vi "UT_011_Comments.vi"() -> ()   [LabVIEW 2017]
uses:
  88135e47-21b0-4fd1-85e0-e7ee9c587d2f.vi
  lib/TOML to LabVIEW.vi
  <vilib>/addons/_JKI Toolkits/Caraya/classes/Assert/Assert True.vi
  <vilib>/addons/_JKI Toolkits/Caraya/classes/Test/Test.lvclass
  <vilib>/addons/_JKI Toolkits/Caraya/classes/Assert/Assert.lvclass
  lib/TOML.lvlib
panel:
  out "error out":errorcluster
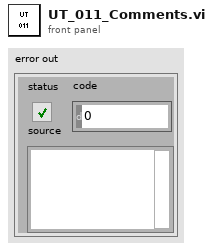
[diagram p1: front panel]
types:
  T1 = typedef "TOML.lvlib/TOML Value.ctl" = cluster{"type":enum16{"Table", "Array", "String", "Integer", "Float", "Boolean", "Offset Date-Time", "Local Date-Time", "Local Date", "Local Time", "Path"}, "value":variant}
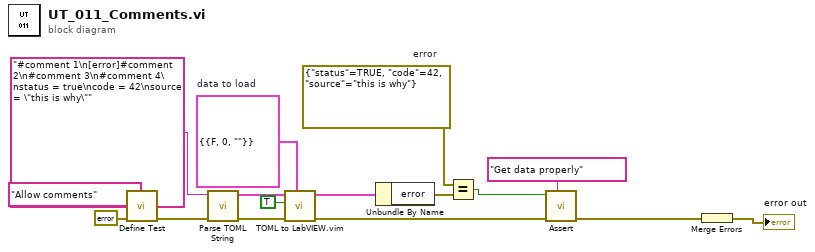
[diagram p0: block diagram]
diagram:
  w7 = cluster{"error":errorcluster} {"error"={"status"=FALSE, "code"=0, "source"=""}}  # data to load
  w9 = errorcluster {"status"=TRUE, "code"=42, "source"="this is why"}  # error
  n1 = call <vilib>:"Define Test.vi"("error in (no error)"=errorcluster {"status"=FALSE, "code"=0, "source"=""}, "Label (VI Title)"="Allow comments") -> ("error out"=w8:errorcluster)  [unwired: 9 in]
  n2 = call "Parse TOML String.vi"("error in (no error)"=w8, "String"="#comment 1\n[error]#comment 2\n#comment 3\n#comment 4\nstatus = true\ncode = 42\nsource = \"this is why\"") -> ("error out"=w2:errorcluster, "Value"=w3:T1)  [unwired: 8 in]
  n3 = call "TOML to LabVIEW.vim"("datatype"=w7, "error in (no error)"=w2, "Error if missing element"=TRUE, "Value"=w3) -> ("error out"=w6:errorcluster, "LV Data"=w4:cluster{"error":errorcluster})  [unwired: 5 in, 1 out]
  n4 = Unbundle By Name(w4) -> ("error"=w10:errorcluster)
  n5 = Equal?(x=w9, y=w10) -> (x = y?=w12:bool)
  n6 = call-poly <vilib>:"Assert.vi"("Label"="Get data properly" ("Label (VI Title)"), "error in (no error)"=w6, "True?"=w12) -> ("error out"=w15:errorcluster)  [unwired: 8 in]
  n7 = Merge Errors(w15) -> (→"error out":errorcluster)
